vi "Dashboard Main.vi"() -> ()   [LabVIEW 2016]
uses:
  <vilib>/Utility/miscctls.llb/LVRowAndColumnTypeDef.ctl
  <vilib>/event_ctls.llb/eventvkey.ctl
  <vilib>/Rock Robotics/Network Tables/NT Read Numeric Array.vi
  <vilib>/Rock Robotics/Network Tables/NT Write String Array.vi
  <vilib>/Rock Robotics/Network Tables/NT Write Numeric Array.vi
  <vilib>/Rock Robotics/WPI/Dashboard/WPI_DashboardLogging Global.vi
panel:
  in  "Camera Settings Right":T1={"Frame Rate"=30, "Compression"=30, "Size"=1, "DB Camera Config"=FALSE} {"Frame Rate" scale=1.0..30.0; "Compression" scale=100.0..-1.0; "Size" items=["640x480", "320x240", "160x120"]}
  in  "Camera Name Right":string(combo)="No Camera Selection"
  out "Camera Info":cluster{"Mbps LED":bool, "Mbps":dbl, "fps":dbl} {"fps" format="%#.1g"; "Mbps" format="%#.1g"}
  in  "Camera Settings":T1={"Frame Rate"=30, "Compression"=30, "Size"=1, "DB Camera Config"=FALSE} {"Frame Rate" scale=1.0..30.0; "Compression" scale=100.0..-1.0; "Size" items=["640x480", "320x240", "160x120"]}
  in  "TCP":refnum<k5>
  in  "Rec Mode":enum32{"Stop", "Record", "Playback"}(radio)
  out "Robot IP":string
  out "Image Message":string="Timeout in Camera Communications"
  in  "Dashboard Tab":T2(tab)
  in  "Select Auto":string(combo)="Select Autonomous ..."
  out "NT Connection":bool
  out "MotorChart R":cluster{"Numeric":dbl, "Numeric":dbl}(graph)
  out "MotorChart L":cluster{"Numeric":dbl, "Numeric":dbl}(graph)
  out "MotorSliders R":cluster{"MotorSlide1":dbl, "MotorSlide2":dbl} {"MotorSlide2" scale=-1.0..1.0 scale format="%#_2e"; "MotorSlide1" scale=-1.0..1.0 scale format="%#_2e"}
  out "MotorSliders L":cluster{"MotorSlide1":dbl, "MotorSlide2":dbl} {"MotorSlide2" scale=-1.0..1.0 scale format="%#_2e"; "MotorSlide1" scale=-1.0..1.0 scale format="%#_2e"}
  out "Gyro":dbl(knob) scale=0.0..360.0
  out "JS1 Z":dbl(slide) scale=-1.0..1.0 scale format="%#_2e"
  out "JS1 Graph":cluster{"X":dbl, "Y":dbl}[](graph)
  out "JS1 Buttons":T3
  out "JS2 Z":dbl(slide) scale=-1.0..1.0 scale format="%#_2e"
  out "JS2 Graph":cluster{"X":dbl, "Y":dbl}[](graph)
  out "JS2 Buttons":T3
  out "Mode":T4(ring)=enum."Auto Disabled"
  out "Camera Image Right":T5(plugin-control)
  in  "DB/String 9":string
  in  "DB/String 8":string
  in  "DB/String 7":string
  in  "DB/String 6":string
  in  "DB/String 5":string
  in  "DB/String 4":string
  in  "DB/String 3":string
  in  "DB/String 2":string
  in  "DB/String 1":string
  in  "DB/String 0":string
  in  "DB/Slider 0":dbl(slide) scale=0.0..5.0
  in  "DB/Slider 1":dbl(slide) scale=0.0..5.0
  in  "DB/Slider 2":dbl(slide) scale=0.0..5.0
  in  "DB/Slider 3":dbl(slide) scale=0.0..5.0
  out "DB/LED 3":bool
  out "DB/LED 2":bool
  out "DB/LED 1":bool
  out "DB/LED 0":bool
  in  "DB/Button 3":bool
  in  "DB/Button 2":bool
  in  "DB/Button 1":bool
  in  "DB/Button 0":bool caption="New Name"
  in  "Path":path
  in  "Test Slider":dbl(slide) scale=0.0..100.0 scale format="%#_3g"
  in  "On/Off":bool caption="Solenoid"
  in  "Test Name":u16(ring) items=["Select the test to run..."]
  in  "Test Tree":string(tree)
  in  "Motor":cluster{"Value":dbl, "Enable":bool} {"Value" scale=-1.0..1.0 scale format="%#_3g"}
  out "Progress":T6 {"Test Progress" scale=0.0..100.0}
  in  "Rev/Fwd":cluster{"Forward":bool, "Reverse":bool}
  in  "Test Ring":u16(ring) items=["Monochrome", "Color"]
  out "Cmd Status":string
  in  "Execute Command":bool
  in  "Command Params":string[][](table)
  in  "Command Selection":i32(listbox)
  in  "CheckList":i32(listbox)
  out "Tree":string(tree)
  out "Camera Image":T5(plugin-control)
  out "Background":bool
  in  "Camera Name":string(combo)="No Camera Selection"
  # "HW"
  # "HW"
  # "Joysticks"
  # "Drive Motors"
  # "Front"
  # "Right"
  # "Left"
  # "Back"
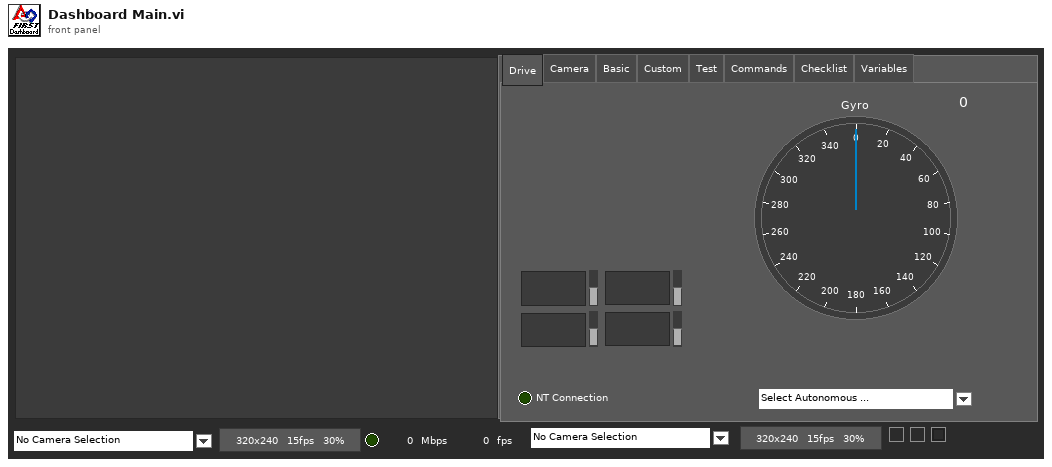
[diagram p1: front panel]
types:
  T1 = cluster{"Frame Rate":i32, "Compression":i32, "Size":u16, "DB Camera Config":bool}
  T2 = enum32{"Drive", "Camera", "Basic", "Custom", "Test", "Commands", "Checklist", "Variables"}
  T3 = cluster{bool, bool, bool, bool, bool, bool, bool, bool, bool, bool, bool, bool}
  T4 = enum8{"Tele-Op Disabled", "Tele-Op Enabled", "Auto Disabled", "Auto Enabled", "Test Disabled", "Test Enabled", "Disconnected", "No Code", "E-Stop"}
  T5 = typedef "IMAQ Image.ctl" = refnum<image>
  T6 = cluster{"Test Progress":u8, "Test Progress Text":string}
  T7 = typedef "Image Type" = u32
  T8 = cluster{"IDs":cluster{"RPC field ID":u16, "Unique ID":u16}, "String":string}
  T9 = enum32{"Drive", "Basic", "Custom", "Test", "Checklist", "Variables"}
  T10 = cluster{"Camera Image":refnum<vi>, "Dashboard Tab":refnum<vi>, "Background":refnum<vi>, "Rec Mode":refnum<vi>, "Test Slider":refnum<vi>, "On/Off ":refnum<vi>, "Test Ring":refnum<vi>, "Rev/Fwd":refnum<vi>, "Test Name":refnum<vi>, "Motor":refnum<vi>, "Progress":refnum<vi>, "CheckList":refnum<vi>, "Tree":refnum<vi>, "Test Tree":refnum<vi>, "Command Params":refnum<vi>, "Command Selection":refnum<vi>, "Execute Command":refnum<vi>, "Cmd Status":refnum<vi>, "Camera Settings":refnum<vi>, "Camera Name":refnum<vi>, "Camera Info":refnum<vi>}
  T11 = cluster{"Error Strings":string, "Disable Counts":cluster{u16, u16}, "Rail Faults":cluster{u16, u16, u16}, "Robot IP":string, "DB Mode":u8, "Event Info":cluster{"Name":string, "Type":u8, "Number":u16, "Replay":u8}}
  T12 = cluster{"Storage":cluster{"Disk Free":u64, "RAM Block":u32, "RAM free":u32}, "CPU Utilization":cluster{"CPU % ISR":sgl, "CPU % Time Crit":sgl, "CPU % Timed Str":sgl, "CPU % High":sgl, "CPU % Above":sgl, "CPU % Normal":sgl, "CPU % Low":sgl}, "CAN":cluster{"% Bus Utilization":sgl, "Bus Off Cnt":u32, "TX_FIFO Full Cnt":u32, "Receive Error Cnt":u8, "Transmit Error Cnt":u8}, "HID":cluster{"HID Outputs":u32, "Rumble Low":u16, "Rumble High":u16}[]}
  T13 = cluster{"Status bits":cluster{"Test Mode":bool, "Autonomous":bool, "Enabled":bool, "Code Start":bool, "Brownout":bool, "Reserved 2":bool, "Reserved 3":bool, "E-Stop":bool}, "Code Trace":cluster{"Disabled":bool, "TeleOp":bool, "Auto":bool, "Test":bool}, "Controller Type":enum16{"unknown", "cRIO", "roboRio"}, "Code?":enum16{"unknown", "noCode", "code"}, "Battery V":dbl}
  T14 = cluster{"Control Bits":cluster{"TestMode":bool, "Autonomous":bool, "Enabled":bool, "FMS Present":bool, bool, bool, bool, "E-Stop":bool}, "Team Station ":u8, "Countdown":sgl, "Joystick Values":cluster{"Axes":dbl[], "Buttons":bool[], "POVs":i16[]}[]}
  T15 = cluster{"Axes":dbl[], "Buttons":bool[], "POVs":i16[]}[]
  T16 = cluster{"Axes":dbl[], "Buttons":bool[], "POVs":i16[]}
  T17 = cluster{"Buttons[0]":bool, "Buttons[1]":bool, "Buttons[2]":bool, "Buttons[3]":bool, "Buttons[4]":bool, "Buttons[5]":bool, "Buttons[6]":bool, "Buttons[7]":bool, "Buttons[8]":bool, "Buttons[9]":bool, "Buttons[10]":bool, "Buttons[11]":bool}
  T18 = cluster{"Operation":enum16{"Update", "Clear"}, "Color Box":u32}[]
  T19 = typedef "eventvkey.ctl" = enum16{"ASCII", "Enter", "Return", "Shift", "Ctrl", "Alt", "Cmd", "Opt", "Caps", "NumLock", "Clear", "Break", "Up", "Down", "Left", "Right", "Insert", "Delete", "Home", "End", "PageUp", "PageDown", "Escape", "Help", "Pause", "ScrollLock", "F1", "F2", "F3", "F4", "F5", "F6", "F7", "F8", "F9", "F10", "F11", "F12", "F13", "F14", "F15", "F16", "F17", "F18", "F19", "F20", "F21", "F22", "F23", "F24", "Play", "VolumeUp", "VolumeDown", "Mute", "Two Byte Char"}
  T20 = cluster{"Image Size":bool, "Image Type":bool, "Pixel Value":bool, "ROI Information":bool, "Zoom Factor":bool}
  T21 = cluster{"Operation":enum16{"Update", "Clear"}, "Color Box":u32}
  T22 = typedef "LVRowAndColumnTypeDef.ctl" = cluster{"Row":i32, "Column":i32}
  T23 = cluster{"Shift":bool, "Ctrl":bool, "Alt":bool, "Cmd":bool, "Opt":bool}
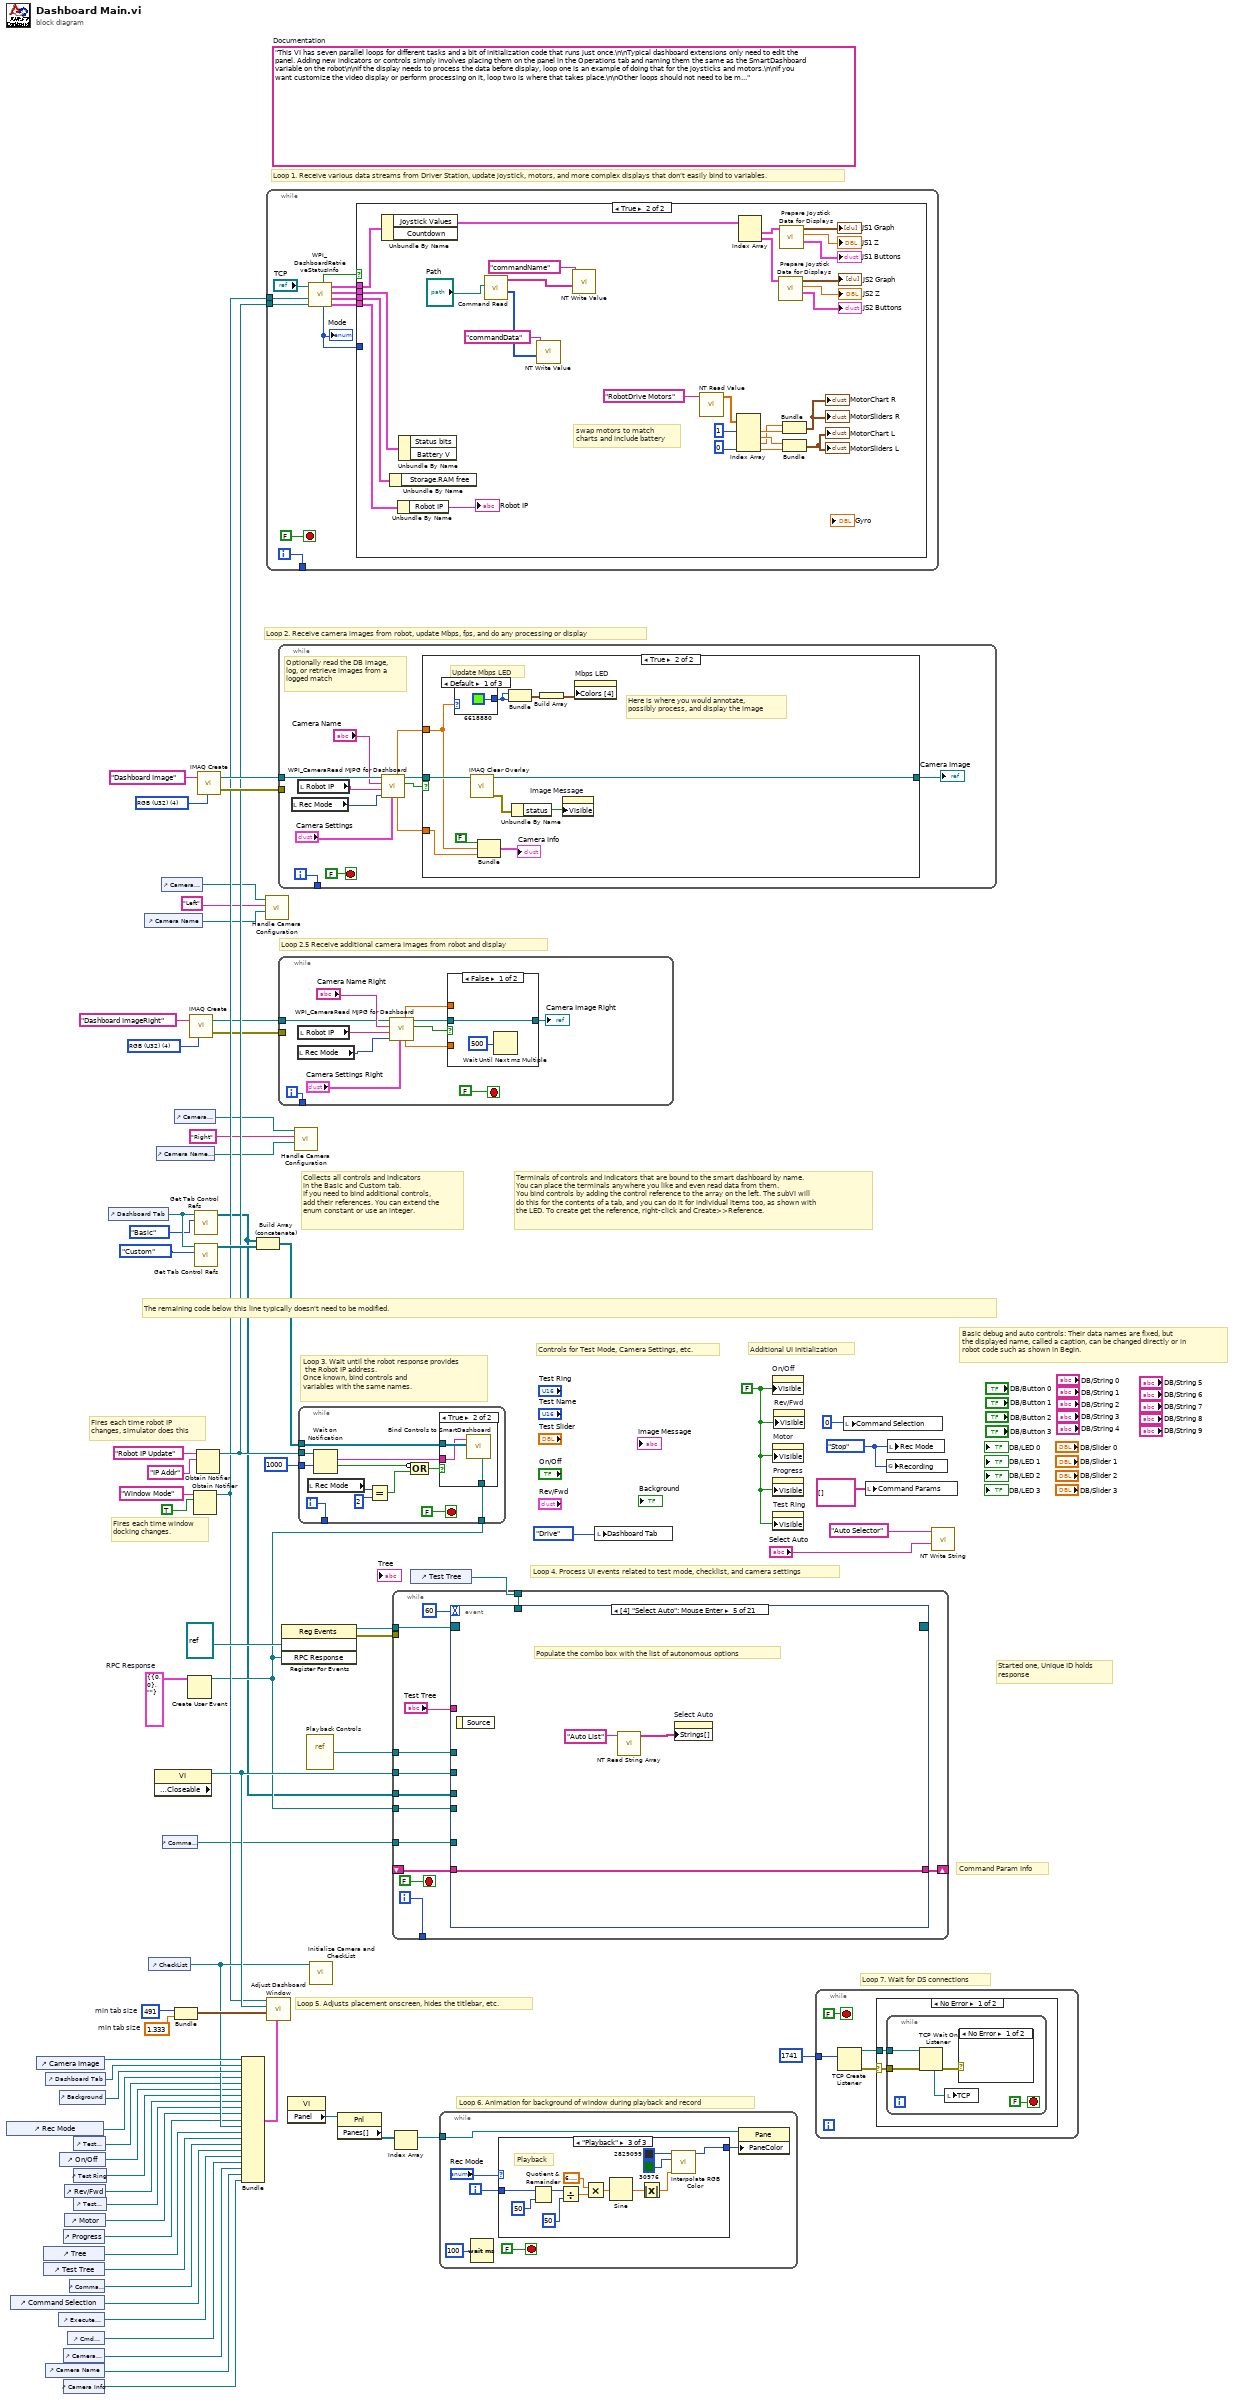
[diagram p0: block diagram]
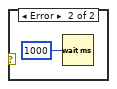
[diagram p3: hidden frame]
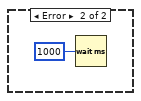
[diagram p4: hidden frame]
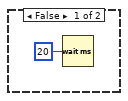
[diagram p5: hidden frame]
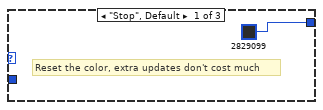
[diagram p6: hidden frame]
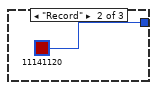
[diagram p7: hidden frame]
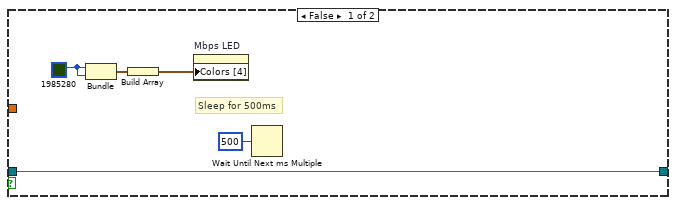
[diagram p9: hidden frame]
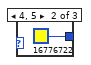
[diagram p10: hidden frame]
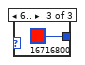
[diagram p11: hidden frame]
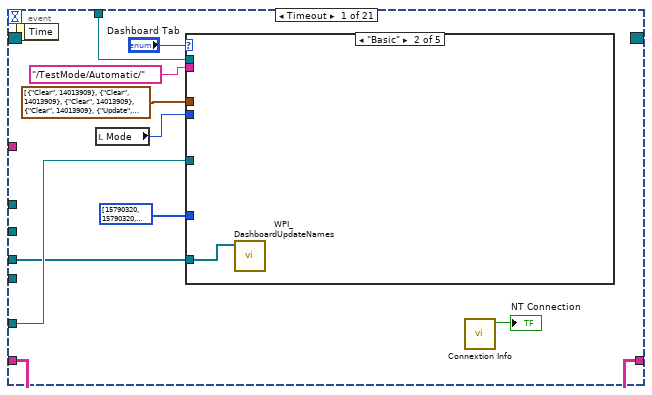
[diagram p12: hidden frame]
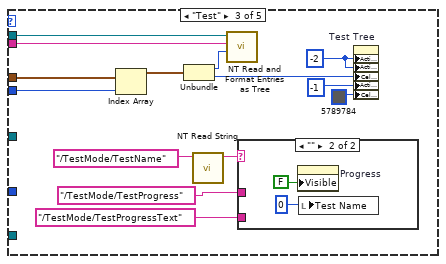
[diagram p14: hidden frame]
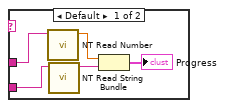
[diagram p15: hidden frame]
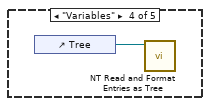
[diagram p16: hidden frame]
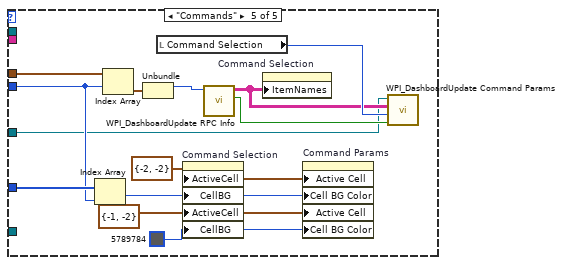
[diagram p17: hidden frame]
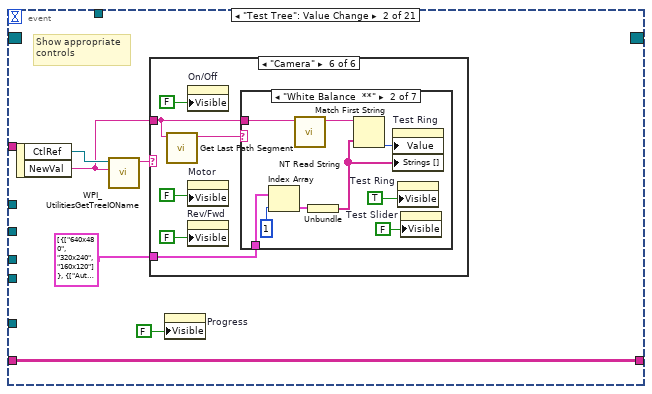
[diagram p18: hidden frame]
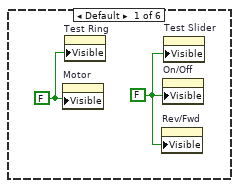
[diagram p19: hidden frame]
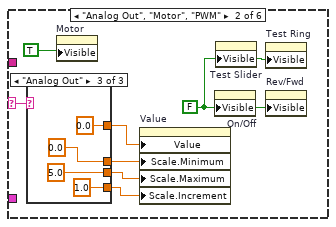
[diagram p20: hidden frame]
diagram:
  w7 = T7 4 items=["Grayscale (U8)", "Grayscale (I16)", "Grayscale (SGL)", "Complex (CSG)", "RGB (U32)", "HSL (U32)", "RGB (U64)"] ("Image Type")
  w23 = T8 {"IDs"={"RPC field ID"=0, "Unique ID"=0}, "String"=""}  # RPC Response
  w48 = 491  # min tab size
  w47 = 1.333  # min tab size
  w55 = enum32{"Stop", "Record", "Playback"}."Stop" ("Rec Mode")
  w30 = FALSE ("Visible")
  (unwired) "This VI has seven parallel loops for different tasks and a bit of initialization code that runs just once.\n\nTypical dashboard extensions only need to edit the panel. Adding new indicators or controls simply involves placing them on the panel in the Operations tab and naming them the same as the SmartDashboard variable on the robot\n\nIf the display needs to process the data before display, loop one is an example of doing that for the joysticks and motors.\n\nIf you want customize the video display or perform processing on it, loop two is where that takes place.\n\nOther loops should not need to be modified. They are pretty standard, and document the task they perform."  # Documentation
  w72 = T7 4 items=["Grayscale (U8)", "Grayscale (I16)", "Grayscale (SGL)", "Complex (CSG)", "RGB (U32)", "HSL (U32)", "RGB (U64)"] ("Image Type")
  # "Loop 2.5 Receive additional camera images from robot and display"
  # "Command Param Info"
  # "Started one, Unique ID holds\nresponse"
  # "Loop 7. Wait for DS connections"
  # "Basic debug and auto controls: Their data names are fixed, but\nthe displayed name, called a caption, can be changed directly or in\nrobot code such as shown in Begin."
  # "Controls for Test Mode, Camera Settings, etc."
  # "Additional UI Initialization"
  # "Loop 6. Animation for background of window during playback and record"
  # "Fires each time robot IP\nchanges, simulator does this"
  # "Fires each time window\ndocking changes."
  # "Collects all controls and indicators\nin the Basic and Custom tab.\nIf you need to bind additional controls,\nadd their references. You can extend the\nenum constant or use an integer."
  # "The remaining code below this line typically doesn't need to be modified."
  # "Loop 4. Process UI events related to test mode, checklist, and camera settings"
  # "Terminals of controls and indicators that are bound to the smart dashboard by name.\nYou can place the terminals anywhere you like and even read data from them.\nYou bind controls by adding the control reference to the array on the left. The subVI will\ndo this for the contents of a tab, and you can do it for individual items too, as shown with\nthe LED. To create get the reference, right-click and Create>>Reference."
  # "Loop 3. Wait until the robot response provides\n the Robot IP address.\nOnce known, bind controls and\nvariables with the same names."
  # "Loop 5. Adjusts placement onscreen, hides the titlebar, etc."
  # "Loop 1. Receive various data streams from Driver Station, update joystick, motors, and more complex displays that don't easily bind to variables."
  # "Loop 2. Receive camera images from robot, update Mbps, fps, and do any processing or display"
  n1 = control-ref of="Rec Mode"() -> (w36:refnum<vi>)
  n2 = control-ref of="Command Selection"() -> (w22:refnum<vi>)
  n3 = control-ref of="Camera Image"() -> (w50:refnum<vi>)
  n4 = control-ref of="Tree"() -> (w40:refnum<vi>)
  n5 = control-ref of="Test Tree"() -> (w39:refnum<vi>)
  n6 = control-ref of="Dashboard Tab"() -> (w49:refnum<vi>)
  n7 = control-ref of="Camera Name"() -> (w13:refnum<vi>)
  n8 = control-ref of="Execute Command"() -> (w24:refnum<vi>)
  n9 = control-ref of="Background"() -> (w45:refnum<vi>)
  n10 = control-ref of="On/Off"() -> (w34:refnum<vi>)
  n11 = control-ref of="Progress"() -> (w31:refnum<vi>)
  n12 = control-ref of="Camera Settings"() -> (w14:refnum<vi>)
  n13 = control-ref of="Camera Info"() -> (w12:refnum<vi>)
  n14 = control-ref of="Rev/Fwd"() -> (w32:refnum<vi>)
  n15 = control-ref of="Motor"() -> (w37:refnum<vi>)
  n16 = control-ref of="Cmd Status"() -> (w18:refnum<vi>)
  n17 = control-ref of="Command Params"() -> (w25:refnum<vi>)
  n18 = control-ref of="Test Slider"() -> (w35:refnum<vi>)
  n19 = control-ref of="Test Ring"() -> (w33:refnum<vi>)
  n20 = control-ref of="Test Name"() -> (w38:refnum<vi>)
  n21 = control-ref of="Dashboard Tab"() -> (w53:refnum<vi>)
  n22 = control-ref of="Camera Name"() -> (w15:refnum<vi>)
  n23 = control-ref of="CheckList"() -> (w41:refnum<vi>)
  n24 = property class="VI" props=["Front Panel.Closeable"]() -> (reference out=w54:refnum<vi>)  [unwired: 2 in, 2 out]
  n25 = control-ref of="Camera Name Right"() -> (w3:refnum<vi>)
  n26 = control-ref of="Camera Settings"() -> (w16:refnum<vi>)
  n27 = control-ref of="Command Params"() -> (w17:refnum<vi>)
  n28 = control-ref of="Camera Settings Right"() -> (w4:refnum<vi>)
  n29 = Bundle("min tab size"=w48, "min tab size"=w47) -> (w46:cluster{"min tab size":i32, "min tab size":dbl})  [unwired: 1 in]
  n30 = Create User Event(user event datatype=w23) -> (user event=w19:refnum<user-event>)  [unwired: 1 in, 1 out]
  n31 = call "IMAQ Create"("Image Name"="Dashboard ImageRight", "Image Type"=w7) -> ("New Image"=w6:T5, "error out"=w5:errorcluster)  [unwired: 2 in, 1 out]
  n32 = Obtain Notifier(name (unnamed)="Window Mode", notification data type=TRUE) -> (notifier out=w28:refnum<notifier>)  [unwired: 2 in, 2 out]
  n33 = call <vilib>:"Get Tab Control Refs.vi"("Page Index"=T9."Basic" ("Dashboard Tab"), "TabControl in"=w53) -> ("ControlsOnPage"=w11:refnum<vi>[])  [unwired: 9 in]
  n34 = call <vilib>:"Get Tab Control Refs.vi"("Page Index"=T9."Custom" ("Dashboard Tab"), "TabControl in"=w53) -> ("ControlsOnPage"=w52:refnum<vi>[])  [unwired: 9 in]
  n35 = Obtain Notifier(name (unnamed)="Robot IP Update", notification data type="IP Addr" ("name (unnamed)")) -> (notifier out=w29:refnum<notifier>)  [unwired: 2 in, 2 out]
  n36 = call "IMAQ Create"("Image Name"="Dashboard Image", "Image Type"=w72) -> ("New Image"=w70:T5, "error out"=w69:errorcluster)  [unwired: 2 in, 1 out]
  n37 = Bundle("Camera Image"=w50, "Dashboard Tab"=w49, "Background"=w45, "Rec Mode"=w36, "Test Slider"=w35, "On/Off"=w34, "Test Ring"=w33, "Rev/Fwd"=w32, "Test Name"=w38, "Motor"=w37, "Progress"=w31, "CheckList"=w41, "Tree"=w40, "Test Tree"=w39, "Command Params"=w25, "Command Selection"=w22, "Execute Command"=w24, "Cmd Status"=w18, "Camera Settings"=w14, "Camera Name"=w13, "Camera Info"=w12) -> (w42:T10)  [unwired: 1 in]
  n38 = Build Array (concatenate)(w11, w52) -> (w51:refnum<vi>[])
  n39 = call "Handle Camera Configuration.vi"("CameraNameRef"=w15, "Camera File Name"="Left", "ClusterRef"=w16) -> ()  [unwired: 9 in]
  n40 = while {
    tunnel: [w82] -> _
    tunnel: w29 -> [w76]
    tunnel: w28 -> [w73]
    i -> [w82]
    stop <- FALSE stop-if-true
    n41 = call <vilib>:"WPI_DashboardRetrieveStatusInfo.vi"("Binding Refnum"=w76, "Window Mode Notifier"=w73, "TCP Cnx"="TCP") -> ("Power and Errors"=w77:T11, "Robot Metrics"=w80:T12, "Status Info"=w81:T13, "Control Info"=w78:T14, "Robot Mode"=w75:T4, "Process?"=w79:bool)  [unwired: 3 in]
    "Mode" <- w75
    n42 = case shown="True" w79 {
      tunnel: w81 -> [_ w113]
      tunnel: w80 -> [_ w112]
      tunnel: w78 -> [_ w111]
      tunnel: w77 -> [_ w110]
      tunnel: w75 -> [_ _]
      frame False {
        n43 = Wait (ms)(milliseconds to wait=u32 20) -> ()  [unwired: 1 out]
      }
      frame True {
        # "swap motors to match\ncharts and include battery"
        n44 = Unbundle By Name(w111) -> ("Joystick Values"=w101:T15)  [unwired: 1 out]
        n45 = Unbundle By Name(w112) -> ()  [unwired: 1 out]
        n46 = Unbundle By Name(w110) -> ("Robot IP"=→"Robot IP":string)
        n47 = Unbundle By Name(w113) -> ()  [unwired: 2 out]
        n48 = call "Command Read.vi"("file path (dialog if empty)"="Path") -> ("value"=w86:i32[], "command"=w88:string[])  [unwired: 9 in]
        n49 = call-poly <vilib>:"NT Write Value.vi"("Numeric Array"=w86, "Name"="commandData") -> ()  [unwired: 9 in, 1 out]
        n50 = call-poly <vilib>:"NT Write Value.vi"("String Array"=w88, "Name"="commandName") -> ()  [unwired: 9 in, 1 out]
        n51 = call-poly <vilib>:"NT Read Value.vi"("Name"="RobotDrive Motors") -> ("Numeric Array"=w91:dbl[])  [unwired: 9 in, 1 out]
        n52 = Index Array(array=w91, index #1=1, index #4=0) -> (element #1=w105:dbl, element #2=w106:dbl, element #3=w104:dbl, element #4=w109:dbl)  [unwired: 2 in]
        n53 = Index Array(array=w101) -> (element #1=w100:T16, element #2=w96:T16)  [unwired: 2 in]
        n54 = call "Prepare Joystick Data for Displays.vi"("Joystick Values"=w96) -> ("Buttons"=→"JS2 Buttons":T17, "Z Axis"=→"JS2 Z":dbl, "Cartesian Data"=→"JS2 Graph":cluster{"X axis":dbl, "X axis":dbl}[])  [unwired: 8 in]
        n55 = call "Prepare Joystick Data for Displays.vi"("Joystick Values"=w100) -> ("Buttons"=→"JS1 Buttons":T17, "Z Axis"=→"JS1 Z":dbl, "Cartesian Data"=→"JS1 Graph":cluster{"X axis":dbl, "X axis":dbl}[])  [unwired: 8 in]
        n56 = Bundle("Numeric"=w104, "Numeric"=w105) -> (→"MotorChart R" →"MotorSliders R":cluster{"Numeric":dbl, "Numeric":dbl})  [unwired: 1 in]
        n57 = Bundle("Numeric"=w106, "Numeric"=w109) -> (→"MotorChart L" →"MotorSliders L":cluster{"Numeric":dbl, "Numeric":dbl})  [unwired: 1 in]
      }
    }
  }
  n58 = call "Adjust Dashboard Window.vi"("Sizing Refnums"=w42, "Size Constraints"=w46, "VI"=w54, "WIn Mode"=w28) -> ()  [unwired: 8 in]
  n59 = while {
    tunnel: w70 -> [w123]
    tunnel: w69 -> [_]
    tunnel: [w124] -> _
    i -> [w124]
    stop <- FALSE stop-if-true
    # "Optionally read the DB image,\nlog, or retrieve images from a\nlogged match"
    n60 = local read "Rec Mode"() -> (w119:enum32{"Stop", "Record", "Playback"})
    n61 = local read "Robot IP"() -> (w118:string)
    n62 = call <vilib>:"WPI_CameraRead MJPG for Dashboard.vi"("Camera Settings"="Camera Settings", "Rec Mode"=w119, "Robot IP"=w118, "Camera Name"="Camera Name", "Refnum in"=w123) -> ("Active"=w121:bool, "Refnum out"=w122:T5, "FPS"=w120:dbl, "Bandwidth (Mbps)"=w117:dbl)  [unwired: 3 in]
    n63 = case shown="True" w121 {
      tunnel: w122 -> [w126 w137]
      tunnel: w117 -> [_ w134]
      tunnel: w120 -> [_ w135]
      tunnel: [w126 w131] -> w114
      frame False {
        w128 = u32 1985280 ("Color Box")
        # "Sleep for 500ms"
        n64 = Bundle("Color Box"=w128, "Color Box"=w128) -> (w129:cluster{"Color Box":u32, "Color Box":u32})  [unwired: 1 out]
        n65 = Build Array(w129) -> (w127:cluster{"Color Box":u32, "Color Box":u32}[])
        n66 = property on="Mbps LED" class="Bool (strict)"("Colors [4]"=w127) -> ()  [unwired: 2 in, 2 out]
        n67 = Wait Until Next ms Multiple(millisecond multiple=u32 500) -> ()  [unwired: 1 out]
      }
      frame True {
        # "Here is where you would annotate,\npossibly process, and display the image"
        # "Update Mbps LED"
        n68 = case shown="Default" w134 {
          tunnel: [u32 6618880 ("Color Box") u32 16776722 ("Color Box") u32 16716800 ("Color Box")] -> w138
          frame Default {
          }
          frame 4, 5 {
          }
          frame 6.. {
          }
        }
        n69 = call "IMAQ Clear Overlay"("Image"=w137) -> ("error out"=w140:errorcluster, "Image Out"=w131:T5)  [unwired: 2 in, 7 out]
        n70 = Bundle(FALSE, "Bandwidth (Mbps)"=w134, "FPS"=w135) -> (→"Camera Info":cluster{bool, "Bandwidth (Mbps)":dbl, "FPS":dbl})  [unwired: 1 in]
        n71 = Bundle("Color Box"=w138, "Color Box"=w138) -> (w139:cluster{"Color Box":u32, "Color Box":u32})  [unwired: 1 out]
        n72 = Unbundle By Name(w140) -> ("status"=w141:bool)
        n73 = Build Array(w139) -> (w136:cluster{"Color Box":u32, "Color Box":u32}[])
        n74 = property on="Image Message" class="Str"("Visible"=w141) -> ()  [unwired: 2 in, 2 out]
        n75 = property on="Mbps LED" class="Bool (strict)"("Colors [4]"=w136) -> ()  [unwired: 2 in, 2 out]
      }
    }
    "Camera Image" <- w114
  }
  n76 = while {
    tunnel: w6 -> [w155]
    tunnel: w5 -> [_]
    tunnel: [w149] -> _
    i -> [w149]
    stop <- FALSE stop-if-true
    n77 = local read "Rec Mode"() -> (w153:enum32{"Stop", "Record", "Playback"})
    n78 = local read "Robot IP"() -> (w154:string)
    n79 = call <vilib>:"WPI_CameraRead MJPG for Dashboard.vi"("Camera Settings"="Camera Settings Right", "Rec Mode"=w153, "Robot IP"=w154, "Camera Name"="Camera Name Right", "Refnum in"=w155) -> ("Active"=w148:bool, "Refnum out"=w151:T5, "FPS"=w146:dbl, "Bandwidth (Mbps)"=w147:dbl)  [unwired: 3 in]
    n80 = case shown="False" w148 {
      tunnel: w151 -> [w157 w159]
      tunnel: w147 -> [_ _]
      tunnel: w146 -> [_ _]
      tunnel: [w157 w159] -> w145
      frame False {
        n81 = Wait Until Next ms Multiple(millisecond multiple=u32 500) -> ()  [unwired: 1 out]
      }
      frame True {
      }
    }
    "Camera Image Right" <- w145
  }
  n82 = register-events(refnum<vi> refnum, w19) -> (reference out=w59:refnum<event-registration>, error out=w58:errorcluster)  [unwired: 2 in]
  n83 = property class="VI"() -> ("Panel"=w62:refnum<vi>)  [unwired: 2 in, 2 out]
  n84 = call "Handle Camera Configuration.vi"("CameraNameRef"=w3, "Camera File Name"="Right", "ClusterRef"=w4) -> ()  [unwired: 9 in]
  n85 = while {
    tunnel: w51 -> [w171]
    tunnel: w29 -> [w169]
    tunnel: [w167] -> _
    tunnel: u32 1000 ("milliseconds to wait") -> [w166]
    tunnel: w19 -> [w160]
    i -> [w167]
    stop <- FALSE stop-if-true
    n86 = local read "Rec Mode"() -> (w162:enum32{"Stop", "Record", "Playback"})
    n87 = Wait on Notification(notifier=w169, timeout in ms (-1)=w166) -> (notification=w168:string, timed out?=w164:bool)  [unwired: 2 in, 2 out]
    n88 = Equal?(x=w162, y=u16 2 ("Rec Mode")) -> (x = y?=w163:bool)
    n89 = Compound Arithmetic op=OR(invert w164, w163) -> (w165:bool)
    n90 = case shown="True" w165 {
      tunnel: w171 -> [_ w174]
      tunnel: w168 -> [_ w173]
      tunnel: w160 -> [_ w172]
      frame False {
      }
      frame True {
        n91 = call <vilib>:"Bind Controls to SmartDashboard.vi"("RPC ref"=w172, "Bound Control Refs"=w174, "Server IP Address"=w173) -> ()  [unwired: 9 in]
      }
    }
  }
  n92 = vi-ref "Playback Controls.vi"() -> (w60:refnum<vi>)
  n93 = call "Initialize Camera and CheckList.vi"("ListBox in"=w41) -> ()  [unwired: 11 in]
  n94 = property class="Pnl"(reference=w62) -> ("Panes[]"=w63:refnum<vi>[])  [unwired: 1 in, 2 out]
  n95 = Index Array(array=w63) -> (element=w61:refnum<vi>)  [unwired: 1 in]
  n96 = control-ref of="Test Tree"() -> (w64:refnum<vi>)
  n97 = while {
    tunnel: [w184] -> _
    tunnel: w64 -> [w183]
    tunnel: w60 -> [w182]
    tunnel: w59 -> [w181]
    tunnel: w58 -> [_]
    tunnel: w54 -> [w180]
    tunnel: w19 -> [w179]
    tunnel: w17 -> [w178]
    shift-right: [w177] -> _
    shift-left: _ -> [w176]
    tunnel: w11 -> [w175]
    i -> [w184]
    stop <- FALSE stop-if-true
    n98 = event shown="[4] \"Select Auto\": Mouse Enter" {
      selector: w181 -> [_ _ _ _ _ _ _ _ _ _ _ _ _ _ _ _ _ _ _ _ _]
      dyn-events: [_ _ _ _ _ _ _ _ _ _ _ _ _ _ _ _ w440 _ _ _ _] -> _
      timeout: u32 60 ("milliseconds to wait") -> [_ _ _ _ _ _ _ _ _ _ _ _ _ _ _ _ _ _ _ _ _]
      tunnel: w183 -> [w196 _ _ _ _ _ _ _ _ _ _ _ _ _ _ _ _ _ _ _ _]
      tunnel: "Test Tree" -> [_ _ _ _ _ _ _ _ _ _ _ w407 w415 w417 w421 w429 _ _ _ _ _]
      tunnel: w182 -> [_ _ _ _ _ _ _ _ _ _ _ _ _ _ _ _ w442 _ w460 _ _]
      tunnel: w180 -> [_ _ _ _ _ _ _ _ _ _ _ _ _ _ _ _ w438 _ _ _ _]
      tunnel: w179 -> [_ _ _ _ _ _ _ _ _ _ _ _ _ _ _ _ w434 _ _ _ _]
      tunnel: w178 -> [w191 _ _ _ _ _ w358 _ _ _ _ _ _ _ _ _ _ _ _ _ _]
      tunnel: [w190 w235 w337 w342 w351 w355 w356 w365 w375 w382 w394 w406 w413 w416 w420 w428 w433 w455 w457 w461 w472] -> w177
      tunnel: w176 -> [w190 w235 w337 w342 w351 w355 w356 _ _ w382 w394 w406 w413 w416 w420 w428 w433 w455 w457 w461 w472]
      tunnel: w175 -> [w188 _ _ _ _ _ _ _ _ _ _ _ _ _ _ _ _ _ _ _ _]
      event Timeout {
        n99 = event-data() -> ()  [unwired: 1 in, 1 out]
        n100 = local read "Mode"() -> (w193:T4)
        n101 = case shown="\"Basic\"" "Dashboard Tab" {
          tunnel: w196 -> [_ _ w212 _ _]
          tunnel: "/TestMode/Automatic/" ("Name Pattern") -> [_ _ w211 _ _]
          tunnel: T18 [{"Operation"=enum."Clear", "Color Box"=14013909}, {"Operation"=enum."Clear", "Color Box"=14013909}, {"Operation"=enum."Clear", "Color Box"=14013909}, {"Operation"=enum."Clear", "Color Box"=14013909}, {"Operation"=enum."Update", "Color Box"=14013909}, {"Operation"=enum."Update", "Color Box"=16777215}, {"Operation"=enum."Clear", "Color Box"=14013909}, {"Operation"=enum."Clear", "Color Box"=14013909}, {"Operation"=enum."Clear", "Color Box"=14013909}] -> [_ _ w204 _ w228]
          tunnel: w193 -> [_ _ w203 _ w227]
          tunnel: u32[] [15790320, 15790320, 15790320, 15790320, 16777215, 16777215, 15790320, 15790320, 15790320] -> [_ _ _ _ w233]
          tunnel: w191 -> [_ _ _ _ w221]
          tunnel: w188 -> [_ w198 _ _ _]
          frame "Custom", Default {
          }
          frame "Basic" {
            n102 = call <vilib>:"WPI_DashboardUpdateNames.vi"("Controls on Tab"=w198) -> ()  [unwired: 11 in]
          }
          frame "Test" {
            w210 = -2 ("Active Item:Row Number")
            n103 = Index Array(array=w204, index=w203) -> (element=w205:T21)
            n104 = Unbundle(w205) -> ("Operation"=w206:enum16{"Update", "Clear"}, "Color Box"=w207:u32)
            n105 = call <vilib>:"NT Read String.vi"("Name"="/TestMode/TestName") -> ("String"=w201:string)  [unwired: 9 in, 1 out]
            n106 = call <vilib>:"NT Read and Format Entries as Tree.vi"("Operation"=w206, "Name Pattern"=w211, "Tree Refnum"=w212) -> ()  [unwired: 7 in, 2 out]
            n107 = case shown="\"\"" w201 {
              tunnel: "/TestMode/TestProgress" ("Name") -> [w214 _]
              tunnel: "/TestMode/TestProgressText" ("Name") -> [w213 _]
              frame Default {
                n108 = call <vilib>:"NT Read Number.vi"("Name"=w214) -> ("Numeric"=w215:dbl)  [unwired: 9 in, 1 out]
                n109 = call <vilib>:"NT Read String.vi"("Name"=w213) -> ("String"=w216:string)  [unwired: 9 in, 1 out]
                n110 = Bundle("Numeric"=w215, "String"=w216) -> (→"Progress":cluster{"Numeric":dbl, "String":string})  [unwired: 1 in]
              }
              frame "" {
                n111 = property on="Progress" class="Clust (strict)"("Visible"=FALSE) -> ()  [unwired: 2 in, 2 out]
                n112 = local write "Test Name"(u16 0) -> ()
              }
            }
            n113 = property on="Test Tree" class="Tree (strict)"("Active Item Row Number"=w210, "ActiveColNum"=w210, "CellBG"=w207, "Active Item Row Number"=-1 ("Active Item:Row Number"), "CellBG"=u32 5789784 ("Color Box")) -> ()  [unwired: 2 in, 2 out]
          }
          frame "Variables" {
            n114 = control-ref of="Tree"() -> (w220:refnum<vi>)
            n115 = call <vilib>:"NT Read and Format Entries as Tree.vi"("Tree Refnum"=w220) -> ()  [unwired: 9 in, 2 out]
          }
          frame "Commands" {
            w229 = u32 5789784 ("Color Box")
            w230 = T22 {"Row"=-1, "Column"=-2} ("Active Cell:Active Cell")
            w232 = T22 {"Row"=-2, "Column"=-2} ("Active Cell:Active Cell")
            n116 = Index Array(array=w233, index=w227) -> (element=w231:u32)
            n117 = Index Array(array=w228, index=w227) -> (element=w226:T21)
            n118 = Unbundle(w226) -> ("Operation"=w225:enum16{"Update", "Clear"})  [unwired: 1 out]
            n119 = local read "Command Selection"() -> (w224:i32)
            n120 = property on="Command Selection" class="MCListbox (strict)"("ActiveCell"=w232, "CellBG"=w231, "ActiveCell"=w230, "CellBG"=w229) -> ()  [unwired: 2 in, 2 out]
            n121 = call <vilib>:"WPI_DashboardUpdate RPC Info.vi"("Operation"=w225) -> ("update"=w223:bool, "commands"=w222:string[][])  [unwired: 9 in]
            n122 = property on="Command Selection" class="MCListbox (strict)"("ItemNames"=w222) -> ()  [unwired: 2 in, 2 out]
            n123 = property on="Command Params" class="Tbl (strict)"("Active Cell"=w232, "Cell BG Color"=w231, "Active Cell"=w230, "Cell BG Color"=w229) -> ()  [unwired: 2 in, 2 out]
            n124 = call <vilib>:"WPI_DashboardUpdate Command Params.vi"("Update"=w223, "NewVal"=w224, "Commands"=w222, "Param Tbl"=w221) -> ()  [unwired: 7 in, 1 out]
          }
        }
        n125 = call <vilib>:"Connextion Info.vi"() -> ("Connected"=→"NT Connection":bool)  [unwired: 10 in, 1 out]
      }
      event "Test Tree": Value Change {
        # "Show appropriate\ncontrols"
        n126 = event-data() -> ("CtlRef"=w238:refnum<vi>, "NewVal"=w236:string)  [unwired: 1 in]
        n127 = call <vilib>:"WPI_UtilitiesGetTreeIOName.vi"("NewVal"=w236, "TreeControl in"=w238) -> ("I/O Name"=w239:string)  [unwired: 9 in]
        n128 = case shown="\"Camera\"" w239 {
          selector: w239 -> [_ w246 _ w268 w277 _]
          tunnel: w236 -> [_ _ w265 w267 _ w284]
          tunnel: cluster{string[]}[] [{["640x480", "320x240", "160x120"]}, {["Auto", "Fixed indoor", "Fixed outdoor 1", "Fixed outdoor 2", "Fixed fluorescent 1", "Fixed fluorescent 2", "Hold current"]}, {["Auto", "Flicker-free 50 Hz", "Flicker-free 60 Hz", "Hold current"]}, {["None", "Prioritize frame rate", "Prioritize image quality"]}, {["Monochrome", "Color"]}] -> [_ _ _ _ _ w283]
          frame Default {
            w241 = FALSE ("Visible")
            w240 = FALSE ("Visible")
            n129 = property on="Motor" class="Clust (strict)"("Visible"=w240) -> ()  [unwired: 2 in, 2 out]
            n130 = property on="Test Ring" class="Ring (strict)"("Visible"=w240) -> ()  [unwired: 2 in, 2 out]
            n131 = property on="Rev/Fwd" class="Clust (strict)"("Visible"=w241) -> ()  [unwired: 2 in, 2 out]
            n132 = property on="On/Off" class="Bool (strict)"("Visible"=w241) -> ()  [unwired: 2 in, 2 out]
            n133 = property on="Test Slider" class="Slide (strict)"("Visible"=w241) -> ()  [unwired: 2 in, 2 out]
          }
          frame "Analog Out", "Motor", "PWM" {
            w247 = FALSE ("Visible")
            n134 = case shown="\"Analog Out\"" w246 {
              tunnel: [1.0 ("Value") -1.0 ("Value") 0.0 ("Value")] -> w245
              tunnel: [255.0 ("Value") 1.0 ("Value") 5.0 ("Value")] -> w244
              tunnel: [128.0 ("Value") 0.0 ("Value") 0.0 ("Value")] -> w243
              tunnel: [64.0 ("Value") 0.5 ("Value") 1.0 ("Value")] -> w242
              frame "PWM" {
              }
              frame "Motor", Default {
              }
              frame "Analog Out" {
              }
            }
            n135 = property on="Motor" class="Clust (strict)"("Visible"=TRUE) -> ()  [unwired: 2 in, 2 out]
            n136 = property on="Value" class="Slide (strict)"("Value"=w243, "Scale.Minimum"=w245, "Scale.Maximum"=w244, "Scale.Increment"=w242) -> ()  [unwired: 2 in, 2 out]
            n137 = property on="On/Off" class="Bool (strict)"("Visible"=w247) -> ()  [unwired: 2 in, 2 out]
            n138 = property on="Test Slider" class="Slide (strict)"("Visible"=w247) -> ()  [unwired: 2 in, 2 out]
            n139 = property on="Test Ring" class="Ring (strict)"("Visible"=w247) -> ()  [unwired: 2 in, 2 out]
            n140 = property on="Rev/Fwd" class="Clust (strict)"("Visible"=w247) -> ()  [unwired: 2 in, 2 out]
          }
          frame "Servo" {
            w263 = FALSE ("Visible")
            n141 = call <vilib>:"NT Read Number.vi"("Name"=w265) -> ("Numeric"=w264:dbl)  [unwired: 9 in, 1 out]
            n142 = property on="Test Slider" class="Slide (strict)"("Visible"=TRUE, "Scale.Maximum"=170.0 ("Scale.Range:Maximum")) -> ()  [unwired: 2 in, 2 out]
            n143 = local write "Test Slider"(w264) -> ()
            n144 = property on="Motor" class="Clust (strict)"("Visible"=w263) -> ()  [unwired: 2 in, 2 out]
            n145 = property on="Rev/Fwd" class="Clust (strict)"("Visible"=w263) -> ()  [unwired: 2 in, 2 out]
            n146 = property on="On/Off" class="Bool (strict)"("Visible"=w263) -> ()  [unwired: 2 in, 2 out]
            n147 = property on="Test Ring" class="Ring (strict)"("Visible"=w263) -> ()  [unwired: 2 in, 2 out]
          }
          frame "Relay", "Solenoid" {
            w266 = FALSE ("Visible")
            n148 = property on="Motor" class="Clust (strict)"("Visible"=w266) -> ()  [unwired: 2 in, 2 out]
            n149 = property on="Test Slider" class="Slide (strict)"("Visible"=w266) -> ()  [unwired: 2 in, 2 out]
            n150 = Search and Replace String(input string=w267, search string="/Value  **", replace string="/Direction") -> (result string=w273:string)  [unwired: 5 in, 3 out]
            n151 = property on="Test Ring" class="Ring (strict)"("Visible"=w266) -> ()  [unwired: 2 in, 2 out]
            n152 = call <vilib>:"NT Read String.vi"("Name"=w273) -> ("String"=w271:string)  [unwired: 9 in, 1 out]
            n153 = Equal?(x="Both directions", y=w271) -> (x = y?=w269:bool)
            n154 = Not(x=w269) -> (.not. x?=w270:bool)
            n155 = property on="Rev/Fwd" class="Clust (strict)"("Visible"=w269) -> ()  [unwired: 2 in, 2 out]
            n156 = property on="On/Off" class="Bool (strict)"("Visible"=w270, "Caption.Text"=w268) -> ()  [unwired: 2 in, 2 out]
          }
          frame "Compressor", "Digital Out" {
            w276 = FALSE ("Visible")
            # "Get direction and finish"
            n157 = property on="Motor" class="Clust (strict)"("Visible"=w276) -> ()  [unwired: 2 in, 2 out]
            n158 = property on="Test Slider" class="Slide (strict)"("Visible"=w276) -> ()  [unwired: 2 in, 2 out]
            n159 = property on="Test Ring" class="Ring (strict)"("Visible"=w276) -> ()  [unwired: 2 in, 2 out]
            n160 = property on="On/Off" class="Bool (strict)"("Visible"=TRUE, "Caption.Text"=w277) -> ()  [unwired: 2 in, 2 out]
            n161 = property on="Rev/Fwd" class="Clust (strict)"("Visible"=FALSE) -> ()  [unwired: 2 in, 2 out]
          }
          frame "Camera" {
            n162 = call <vilib>:"Get Last Path Segment.vi"("String in"=w284) -> ("String out"=w285:string)  [unwired: 10 in]
            n163 = property on="On/Off" class="Bool (strict)"("Visible"=FALSE) -> ()  [unwired: 2 in, 2 out]
            n164 = property on="Motor" class="Clust (strict)"("Visible"=FALSE) -> ()  [unwired: 2 in, 2 out]
            n165 = property on="Rev/Fwd" class="Clust (strict)"("Visible"=FALSE) -> ()  [unwired: 2 in, 2 out]
            n166 = case shown="\"White Balance  **\"" w285 {
              tunnel: w284 -> [w291 w300 w309 w318 w327 _ w333]
              tunnel: w283 -> [w289 w297 w306 w315 w324 _ _]
              frame "Size  **" {
                n167 = Index Array(array=w289) -> (element=w288:cluster{string[]})  [unwired: 1 in]
                n168 = call <vilib>:"NT Read String.vi"("Name"=w291) -> ("String"=w290:string)  [unwired: 9 in, 1 out]
                n169 = Unbundle(w288) -> (w286:string[])
                n170 = Match First String(2:w286, 3:w290) -> (0:w287:i32)  [unwired: 1 out]
                n171 = property on="Test Ring" class="Ring (strict)"("Value"=w287, "Strings []"=w286) -> ()  [unwired: 2 in, 2 out]
                n172 = property on="Test Ring" class="Ring (strict)"("Visible"=TRUE) -> ()  [unwired: 2 in, 2 out]
                n173 = property on="Test Slider" class="Slide (strict)"("Visible"=FALSE) -> ()  [unwired: 2 in, 2 out]
              }
              frame "White Balance  **" {
                n174 = Index Array(array=w297, index=1) -> (element=w298:cluster{string[]})
                n175 = call <vilib>:"NT Read String.vi"("Name"=w300) -> ("String"=w299:string)  [unwired: 9 in, 1 out]
                n176 = Unbundle(w298) -> (w295:string[])
                n177 = Match First String(2:w295, 3:w299) -> (0:w294:i32)  [unwired: 1 out]
                n178 = property on="Test Ring" class="Ring (strict)"("Value"=w294, "Strings []"=w295) -> ()  [unwired: 2 in, 2 out]
                n179 = property on="Test Ring" class="Ring (strict)"("Visible"=TRUE) -> ()  [unwired: 2 in, 2 out]
                n180 = property on="Test Slider" class="Slide (strict)"("Visible"=FALSE) -> ()  [unwired: 2 in, 2 out]
              }
              frame "Exposure  **" {
                n181 = Index Array(array=w306, index=2) -> (element=w307:cluster{string[]})
                n182 = call <vilib>:"NT Read String.vi"("Name"=w309) -> ("String"=w308:string)  [unwired: 9 in, 1 out]
                n183 = Unbundle(w307) -> (w303:string[])
                n184 = Match First String(2:w303, 3:w308) -> (0:w304:i32)  [unwired: 1 out]
                n185 = property on="Test Ring" class="Ring (strict)"("Value"=w304, "Strings []"=w303) -> ()  [unwired: 2 in, 2 out]
                n186 = property on="Test Ring" class="Ring (strict)"("Visible"=TRUE) -> ()  [unwired: 2 in, 2 out]
                n187 = property on="Test Slider" class="Slide (strict)"("Visible"=FALSE) -> ()  [unwired: 2 in, 2 out]
              }
              frame "Exposure Priority  **" {
                n188 = Index Array(array=w315, index=3) -> (element=w316:cluster{string[]})
                n189 = call <vilib>:"NT Read String.vi"("Name"=w318) -> ("String"=w317:string)  [unwired: 9 in, 1 out]
                n190 = Unbundle(w316) -> (w312:string[])
                n191 = Match First String(2:w312, 3:w317) -> (0:w313:i32)  [unwired: 1 out]
                n192 = property on="Test Ring" class="Ring (strict)"("Value"=w313, "Strings []"=w312) -> ()  [unwired: 2 in, 2 out]
                n193 = property on="Test Ring" class="Ring (strict)"("Visible"=TRUE) -> ()  [unwired: 2 in, 2 out]
                n194 = property on="Test Slider" class="Slide (strict)"("Visible"=FALSE) -> ()  [unwired: 2 in, 2 out]
              }
              frame "Color Enable  **" {
                n195 = Index Array(array=w324, index=4) -> (element=w325:cluster{string[]})
                n196 = call <vilib>:"NT Read String.vi"("Name"=w327) -> ("String"=w326:string)  [unwired: 9 in, 1 out]
                n197 = Unbundle(w325) -> (w321:string[])
                n198 = Match First String(2:w321, 3:w326) -> (0:w322:i32)  [unwired: 1 out]
                n199 = property on="Test Ring" class="Ring (strict)"("Value"=w322, "Strings []"=w321) -> ()  [unwired: 2 in, 2 out]
                n200 = property on="Test Ring" class="Ring (strict)"("Visible"=TRUE) -> ()  [unwired: 2 in, 2 out]
                n201 = property on="Test Slider" class="Slide (strict)"("Visible"=FALSE) -> ()  [unwired: 2 in, 2 out]
              }
              frame Default {
                n202 = property on="Test Ring" class="Ring (strict)"("Visible"=FALSE) -> ()  [unwired: 2 in, 2 out]
                n203 = property on="Test Slider" class="Slide (strict)"("Visible"=FALSE) -> ()  [unwired: 2 in, 2 out]
              }
              frame "Brightness  **", "Color Level  **", "Compression  **", "FPS  **", "Sharpness  **" {
                n204 = call <vilib>:"NT Read Number.vi"("Name"=w333) -> ("Numeric"=w332:dbl)  [unwired: 9 in, 1 out]
                n205 = local write "Test Slider"(w332) -> ()
                n206 = property on="Test Slider" class="Slide (strict)"("Visible"=TRUE, "Scale.Maximum"=100.0 ("Scale.Range:Maximum")) -> ()  [unwired: 2 in, 2 out]
                n207 = property on="Test Ring" class="Ring (strict)"("Visible"=FALSE) -> ()  [unwired: 2 in, 2 out]
              }
            }
          }
        }
        n208 = property on="Progress" class="Clust (strict)"("Visible"=FALSE) -> ()  [unwired: 2 in, 2 out]
      }
      event "Test Name": Mouse Enter {
        # "Populate the ring with the list of tests"
        n209 = event-data() -> ()  [unwired: 1 in, 1 out]
        n210 = call <vilib>:"NT Read String Array.vi"("Name"="/TestMode/TestList") -> ("String Array"=w341:string[])  [unwired: 9 in, 1 out]
        n211 = Build Array (concatenate)("Select the test to run...", w341) -> (w340:string[])
        n212 = property on="Test Name" class="Ring (strict)"("Strings []"=w340) -> ()  [unwired: 2 in, 2 out]
      }
      event "Test Name": Value Change {
        w343 = FALSE ("Visible")
        # "Tell the robot the test name to run"
        n213 = event-data() -> ("NewVal"=w347:u16)  [unwired: 1 in]
        n214 = property on="Test Name" class="Ring (strict)"() -> ("Strings []"=w348:string[])  [unwired: 2 in, 2 out]
        n215 = local write "Progress"(T6 {"Test Progress"=0, "Test Progress Text"=""} ("Progress")) -> ()
        n216 = Index Array(array=w348, index=w347) -> (element=w346:string)
        n217 = call <vilib>:"NT Write String.vi"("String"=w346, "Name"="/TestMode/TestName") -> ()  [unwired: 9 in, 1 out]
        n218 = property on="Progress" class="Clust (strict)"("Visible"=TRUE) -> ()  [unwired: 2 in, 2 out]
        n219 = property on="Motor" class="Clust (strict)"("Visible"=w343) -> ()  [unwired: 2 in, 2 out]
        n220 = property on="Test Slider" class="Slide (strict)"("Visible"=w343) -> ()  [unwired: 2 in, 2 out]
        n221 = property on="On/Off" class="Bool (strict)"("Visible"=w343) -> ()  [unwired: 2 in, 2 out]
        n222 = property on="Rev/Fwd" class="Clust (strict)"("Visible"=w343) -> ()  [unwired: 2 in, 2 out]
        n223 = property on="Test Ring" class="Ring (strict)"("Visible"=w343) -> ()  [unwired: 2 in, 2 out]
      }
      event "Select Auto": Mouse Enter {
        # "Populate the combo box with the list of autonomous options"
        n224 = event-data() -> ()  [unwired: 1 in, 1 out]
        n225 = call <vilib>:"NT Read String Array.vi"("Name"="Auto List") -> ("String Array"=w350:string[])  [unwired: 9 in, 1 out]
        n226 = property on="Select Auto" class="CmbBox"("Strings[]"=w350) -> ()  [unwired: 2 in, 2 out]
      }
      event "Select Auto": Value Change {
        # "User modified the Auto Selection. Write to NT variable so robot knows."
        n227 = event-data() -> ("NewVal"=w353:string)  [unwired: 1 in]
        n228 = call <vilib>:"NT Write String.vi"("String"=w353, "Name"="Auto Selector") -> ()  [unwired: 9 in, 1 out]
      }
      event "Command Selection": Value Change {
        # "Get the params and show in table"
        n229 = event-data() -> ("NewVal"=w359:i32)  [unwired: 1 in]
        n230 = property on="Command Selection" class="MCListbox (strict)"() -> ("ItemNames"=w357:string[][])  [unwired: 2 in, 2 out]
        n231 = call <vilib>:"WPI_DashboardUpdate Command Params.vi"("NewVal"=w359, "Commands"=w357, "Param Tbl"=w358) -> ()  [unwired: 8 in, 1 out]
      }
      event "Execute Command": Value Change {
        # "Started one, Unique ID holds\nresponse"
        n232 = event-data() -> ()  [unwired: 1 in, 1 out]
        n233 = property on="Command Selection" class="MCListbox (strict)"() -> ("ItemNames"=w370:string[][])  [unwired: 2 in, 2 out]
        n234 = Index Array(array=w370, index (row)="Command Selection", index (col)=0) -> (element=w368:string)
        n235 = call <vilib>:"Invoke Commands.vi"("Command Params"="Command Params", "Function Name"=w368) -> ("Params"=w364:u8, "Started"=w363:bool)  [unwired: 7 in, 1 out]
        n236 = Array Subset(array="Command Params", length (row)=w364) -> (w365:string[][])  [unwired: 3 in]
        n237 = Select(t="Executing" ("Cmd Status"), s=w363, f="" ("Cmd Status")) -> (s? t:f=→"Cmd Status":string)
      }
      event "Command Selection": Double Click {
        n238 = event-data() -> ("Row"=w378:i32)  [unwired: 1 in]
        n239 = property on="Command Selection" class="MCListbox (strict)"() -> ("ItemNames"=w381:string[][])  [unwired: 2 in, 2 out]
        n240 = local read "Command Params"() -> (w377:string[][])
        n241 = Index Array(array=w381, index (row)=w378, index (col)=0) -> (element=w379:string)
        n242 = call <vilib>:"Invoke Commands.vi"("Command Params"=w377, "Function Name"=w379) -> ("Params"=w376:u8, "Started"=w371:bool)  [unwired: 7 in, 1 out]
        n243 = Array Subset(array=w377, length (row)=w376) -> (w375:string[][])  [unwired: 3 in]
        n244 = Select(t="Executing" ("Cmd Status"), s=w371, f="" ("Cmd Status")) -> (s? t:f=w372:string)
        n245 = local write "Cmd Status"(w372) -> ()
      }
      event "CheckList": Double Click {
        # "Shift clears all"
        # "Update symbols on the listbox"
        n246 = event-data() -> ("PlatMods.Shift"=w383:bool, "Row"=w385:i32)  [unwired: 1 in]
        n247 = case shown="True" w383 {
          tunnel: w385 -> [w389 _]
          tunnel: 1 -> [w388 _]
          frame False {
            n248 = property on="CheckList" class="LstBox (strict)"() -> ("Item Symbols"=w387:i32[])  [unwired: 2 in, 2 out]
            n249 = Replace Array Subset(array=w387, new element=w388, index=w389) -> (w386:i32[])
            n250 = property on="CheckList" class="LstBox (strict)"("Item Symbols"=w386) -> ()  [unwired: 2 in, 2 out]
          }
          frame True {
            w390 = 0 ("Top Row")
            n251 = property on="CheckList" class="LstBox (strict)"() -> ("Number of Rows"=w392:u32)  [unwired: 2 in, 2 out]
            n252 = Initialize Array(0, w392) -> (w391:i32[])
            n253 = property on="CheckList" class="LstBox (strict)"("Top Row"=w390, "Value"=w390, "Item Symbols"=w391) -> ()  [unwired: 2 in, 2 out]
          }
        }
      }
      event "CheckList": Key Down {
        # "Update symbols on the listbox\nLeft and right keys check and uncheck"
        n254 = event-data() -> ("VKey"=w396:T19)  [unwired: 1 in]
        n255 = case shown="\"Left\", \"Right\"" w396 {
          selector: w396 -> [w401 _]
          tunnel: eventvkey."Left" ("VKey") -> [w399 _]
          frame "Left", "Right" {
            n256 = Equal?(x=w399, y=w401) -> (x = y?=w400:bool)
            n257 = Select(t=0, s=w400, f=1) -> (s? t:f=w402:i32)
            n258 = property on="CheckList" class="LstBox (strict)"() -> ("Item Symbols"=w405:i32[])  [unwired: 2 in, 2 out]
            n259 = Replace Array Subset(array=w405, new element=w402, index="CheckList") -> (w404:i32[])
            n260 = property on="CheckList" class="LstBox (strict)"("Item Symbols"=w404) -> ()  [unwired: 2 in, 2 out]
          }
          frame Default {
          }
        }
      }
      event "Motor.Enable": Value Change {
        # "When the test mode otor enable helper is set, update that\ntree row item's value"
        n261 = event-data() -> ("NewVal"=w411:bool)  [unwired: 1 in]
        n262 = Unbundle("Motor") -> ("Value"=w410:dbl)  [unwired: 1 out]
        n263 = Select(t=w410, s=w411, f=0.0) -> (s? t:f=w408:dbl)
        n264 = call <vilib>:"NT Write Number.vi"("Numeric"=w408, "Name"=w407) -> ()  [unwired: 9 in, 1 out]
      }
      event "Test Slider": Value Change {
        # "When the test mode slider helper is set, update that\ntree row item's value"
        n265 = event-data() -> ("NewVal"=w414:dbl)  [unwired: 1 in]
        n266 = call <vilib>:"NT Write Number.vi"("Numeric"=w414, "Name"=w415) -> ()  [unwired: 9 in, 1 out]
      }
      event "On/Off": Value Change {
        # "When the test mode on/off helper value is set, update that\ntree row item's value"
        n267 = event-data() -> ("NewVal"=w419:bool)  [unwired: 1 in]
        n268 = Boolean To (0,1)(Boolean=w419) -> (0, 1=w418:i16)
        n269 = call <vilib>:"NT Write Number.vi"("Numeric"=w418, "Name"=w417) -> ()  [unwired: 9 in, 1 out]
      }
      event "Rev/Fwd": Value Change {
        # "When the test mode helper value for relays is set, update that\ntree row item's value"
        n270 = event-data() -> ("NewVal.Forward"=w427:bool, "NewVal.Reverse"=w426:bool)  [unwired: 1 in]
        n271 = Boolean To (0,1)(Boolean=w427) -> (0, 1=w423:i16)
        n272 = Boolean To (0,1)(Boolean=w426) -> (0, 1=w425:i16)
        n273 = Negate(x=w425) -> (-x=w424:i16)
        n274 = Add(x=w423, y=w424) -> (x+y=w422:i16)
        n275 = call <vilib>:"NT Write Number.vi"("Numeric"=w422, "Name"=w421) -> ()  [unwired: 9 in, 1 out]
      }
      event "Test Ring": Value Change {
        # "When a test mode helper value is selected from the ring,\nset the tree item's variable to the string value"
        n276 = event-data() -> ("NewVal"=w431:u16)  [unwired: 1 in]
        n277 = property on="Test Ring" class="Ring (strict)"() -> ("Strings []"=w432:string[])  [unwired: 2 in, 2 out]
        n278 = Index Array(array=w432, index=w431) -> (element=w430:string)
        n279 = call <vilib>:"NT Write String.vi"("String"=w430, "Name"=w429) -> ()  [unwired: 9 in, 1 out]
      }
      event "Rec Mode": Value Change {
        # "Update globals for recording mode and path to read log from.\nClear when logging and let NetworkTables set path for vision to\nuse."
        n280 = event-data() -> ("NewVal"=w443:enum32{"Stop", "Record", "Playback"})  [unwired: 1 in]
        n281 = global write "WPI_DashboardLogging Global.vi" "Logging Filename"(path "") -> ()
        n282 = global write "WPI_DashboardLogging Global.vi" "Recording"(w443) -> ()
        n283 = case shown="\"Playback\"" w443 {
          tunnel: w442 -> [_ w445 w454]
          tunnel: [_ _ w453] -> w440
          tunnel: [_ _ w452] -> _
          tunnel: w438 -> [_ _ w450]
          tunnel: cluster{i32, i32} {-250, 170} -> [_ _ w449]
          tunnel: [_ _ T20 {"Image Size"=TRUE, "Image Type"=TRUE, "Pixel Value"=TRUE, "ROI Information"=TRUE, "Zoom Factor"=FALSE} ("Image Information Shown:All Elements")] -> w436
          tunnel: [_ _ TRUE ("Zoom Factor")] -> w435
          tunnel: w434 -> [_ _ w446]
          frame Default {
          }
          frame "Stop", "Record" {
            # "Place Window too"
            n284 = invoke class="VI" method="FP.Close"(reference=w445) -> (reference out=w444:refnum<vi>)  [unwired: 2 in, 2 out]
            n285 = invoke class="VI" method="Abort VI"(reference=w444) -> ()  [unwired: 2 in, 3 out]
          }
          frame "Playback" {
            n286 = call "Open Playback Panel.vi"("Offset"=w449, "DB VI Ref"=w450, "Playback in"=w454) -> ("Playback out"=w451:refnum<vi>)  [unwired: 8 in]
            n287 = register-events(w451, w446) -> (reference out=w453:refnum<event-registration>, error out=w452:errorcluster)  [unwired: 2 in]
          }
        }
        n288 = property on="Camera Image" class="ImageControl"("Image Information Shown"=w436, "Image Information Visible"=w435) -> ()  [unwired: 2 in, 2 out]
        n289 = call <vilib>:"WPI_DashboardNT Log FieldName Cache.vi"("Operation"=enum16{"Lookup/Add", "Index", "Clear"}."Clear") -> ()  [unwired: 8 in, 3 out]
      }
      event Panel Close {
        w456 = enum32{"Stop", "Record", "Playback"}."Stop" ("Rec Mode")
        # "Playback window has been closed, abort"
        n290 = event-data() -> ()  [unwired: 1 in, 4 out]
        n291 = local write "Rec Mode"(w456) -> ()
        n292 = global write "WPI_DashboardLogging Global.vi" "Recording"(w456) -> ()
      }
      event Panel Close {
        # "Abort playback window and ourself"
        n293 = event-data() -> ()  [unwired: 1 in, 4 out]
        n294 = invoke class="VI" method="FP.Close"(reference=w460) -> (reference out=w459:refnum<vi>)  [unwired: 2 in, 2 out]
        n295 = invoke class="VI" method="Abort VI"(reference=w459) -> (error out=w458:errorcluster)  [unwired: 2 in, 2 out]
        n296 = invoke class="VI" method="Abort VI"(error in=w458) -> ()  [unwired: 2 in, 3 out]
      }
      event User Event {
        n297 = event-data() -> ("IDs"=w467:cluster{"RPC field ID":u16, "Unique ID":u16}, "String"=w466:string)  [unwired: 1 in]
        n298 = Bundle("IDs"=w467, "String"=w466) -> (w465:T8)  [unwired: 1 in]
        n299 = call <vilib>:"Retrieve RPC Response.vi"("RPC Response"=w465) -> ("Output"=w463:string[][])  [unwired: 10 in]
        n300 = Build Array (concatenate)(w461, w463) -> (w462:string[][])
        n301 = local write "Command Params"(w462) -> ()
        n302 = local write "Cmd Status"("" ("Cmd Status")) -> ()
      }
      event "Tree": Double Click {
        n303 = event-data() -> ("PlatMods"=w471:T23, "Tag"=w470:string)  [unwired: 1 in]
        n304 = Unbundle(w471) -> ("Shift"=w469:bool)  [unwired: 4 out]
        n305 = Not(x=w469) -> (.not. x?=w468:bool)
        n306 = call <vilib>:"NT Update Persistence.vi"("Persistence"=w468, "Name"=w470) -> ()  [unwired: 9 in, 1 out]
      }
    }
  }
  n307 = while {
    tunnel: w61 -> [w474]
    i -> [w477]
    stop <- FALSE stop-if-true
    n308 = Wait (ms)(milliseconds to wait=u32 100) -> ()  [unwired: 1 out]
    n309 = case shown="\"Playback\"" "Rec Mode" {
      tunnel: w477 -> [_ _ w492]
      tunnel: [u32 2829099 ("Base Color") u32 11141120 ("Target Color") w481] -> w473
      frame "Stop", Default {
        # "Reset the color, extra updates don't cost much"
      }
      frame "Record" {
      }
      frame "Playback" {
        # "Playback"
        n310 = Quotient & Remainder(x=w492, y=u32 50 ("milliseconds to wait")) -> (x-y*floor(x/y)=w488:u32)  [unwired: 1 out]
        n311 = Divide(x=w488, y=u32 50 ("milliseconds to wait")) -> (x/y=w485:dbl)
        n312 = Multiply(x=6.283185307179586, y=w485) -> (x*y=w490:dbl)
        n313 = Sine(x=w490) -> (sin(x)=w489:dbl)
        n314 = Absolute Value(x=w489) -> (abs(x)=w482:dbl)
        n315 = call "Interpolate RGB Color.vi"("Proportion"=w482, "Target Color"=u32 30976, "Base Color"=u32 2829099) -> ("Result Color"=w481:u32)  [unwired: 8 in]
      }
    }
    n316 = property class="Pane"(reference=w474, "PaneColor"=w473) -> ()  [unwired: 1 in, 2 out]
  }
  n317 = local write "Dashboard Tab"(T2."Drive" ("Dashboard Tab")) -> ()
  n318 = property on="On/Off" class="Bool (strict)"("Visible"=w30) -> ()  [unwired: 2 in, 2 out]
  n319 = property on="Motor" class="Clust (strict)"("Visible"=w30) -> ()  [unwired: 2 in, 2 out]
  n320 = property on="Progress" class="Clust (strict)"("Visible"=w30) -> ()  [unwired: 2 in, 2 out]
  n321 = property on="Test Ring" class="Ring (strict)"("Visible"=w30) -> ()  [unwired: 2 in, 2 out]
  n322 = property on="Rev/Fwd" class="Clust (strict)"("Visible"=w30) -> ()  [unwired: 2 in, 2 out]
  n323 = while {
    tunnel: u16 1741 ("timeout ms (25000)") -> [w494]
    stop <- FALSE stop-if-true
    n324 = TCP Create Listener(10:w494) -> (0:w493:errorcluster, 3:w495:refnum<k5>)  [unwired: 4 in, 1 out]
    n325 = case shown="No Error" w493 {
      selector: w493 -> [w497 _]
      tunnel: w495 -> [w498 _]
      frame No Error {
        n326 = while {
          tunnel: w498 -> [w501]
          tunnel: w497 -> [w500]
          stop <- FALSE stop-if-true
          n327 = TCP Wait On Listener(8:w500, 11:w501) -> (0:w502:errorcluster, 4:w503:refnum<k5>)  [unwired: 2 in, 3 out]
          n328 = local write "TCP"(w503) -> ()
          n329 = case shown="No Error" w502 {
            frame No Error {
            }
            frame Error {
              n330 = Wait (ms)(milliseconds to wait=u32 1000) -> ()  [unwired: 1 out]
            }
          }
        }
      }
      frame Error {
        n331 = Wait (ms)(milliseconds to wait=u32 1000) -> ()  [unwired: 1 out]
      }
    }
  }
  n332 = local write "Command Selection"(u16 0 ("milliseconds to wait")) -> ()
  n333 = local write "Command Params"(string[][] [] ("Command Params")) -> ()
  n334 = global write "WPI_DashboardLogging Global.vi" "Recording"(w55) -> ()
  n335 = local write "Rec Mode"(w55) -> ()
  n336 = call <vilib>:"NT Write String.vi"("String"="Select Auto", "Name"="Auto Selector") -> ()  [unwired: 9 in, 1 out]
